vi "ElevatorManualControl.vi"(9 "Elevator State":string) -> (0 "Manual Contribution":dbl)   [LabVIEW 2018]
uses:
  Inputs_DriverStation.vi
  RobotStates.vi
panel:
  in  "Max Climb Down Power":dbl=0.2
  in  "Max Climb Up Power":dbl=0.6
  in  "Bump Up":dbl=1.0
  in  "Bump Down":dbl=1.0
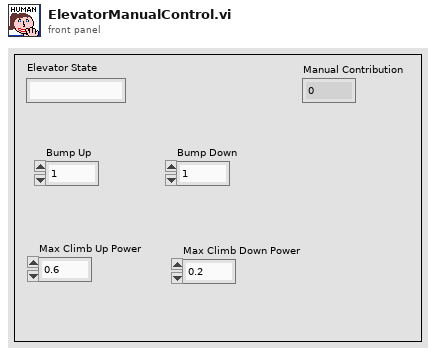
[diagram p1: front panel]
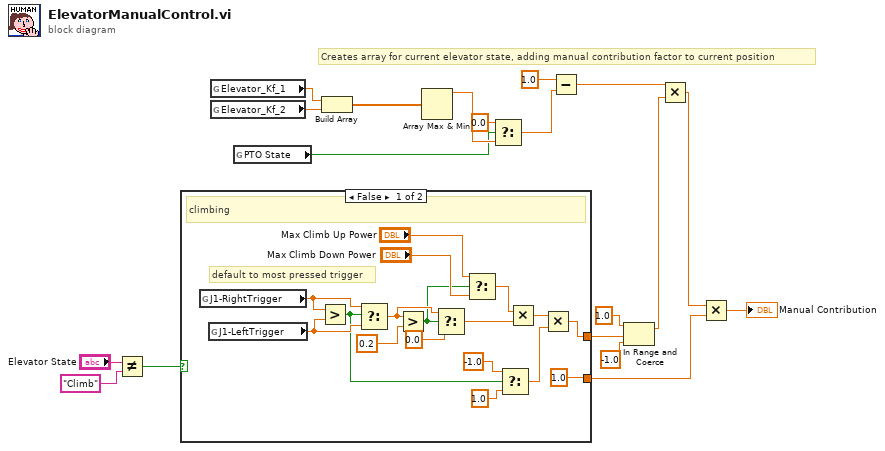
[diagram p0: block diagram]
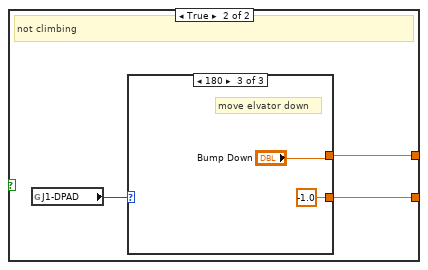
[diagram p2: hidden frame]
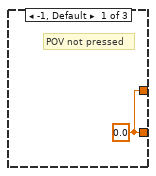
[diagram p3: hidden frame]
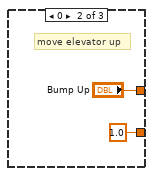
[diagram p4: hidden frame]
diagram:
  # "Creates array for current elevator state, adding manual contribution factor to current position"
  n1 = Not Equal?(x="Elevator State", y="Climb") -> (x != y?=w2:bool)
  n2 = case shown="False" w2 {
    tunnel: [1.0 w39] -> w19
    tunnel: [w23 w38] -> w12
    frame False {
      # "default to most pressed trigger"
      # "climbing"
      n3 = global read "Inputs_DriverStation.vi" "J1-RightTrigger"() -> (w36:dbl)
      n4 = global read "Inputs_DriverStation.vi" "J1-LeftTrigger"() -> (w35:dbl)
      n5 = Greater?(x=w36, y=w35) -> (0:w21:bool)
      n6 = Select(t=w36, s=w21, f=w35) -> (s? t:f=w33:dbl)
      n7 = Greater?(x=w33, y=0.2) -> (0:w27:bool)
      n8 = Select(t=w33, s=w27, f=0.0) -> (s? t:f=w30:dbl)
      n9 = Select(t="Max Climb Up Power", s=w27, f="Max Climb Down Power") -> (s? t:f=w31:dbl)
      n10 = Select(t=-1.0, s=w21, f=1.0) -> (s? t:f=w22:dbl)
      n11 = Multiply(x=w31, y=w30) -> (x*y=w24:dbl)
      n12 = Multiply(x=w24, y=w22) -> (x*y=w23:dbl)
    }
    frame True {
      # "not climbing"
      n13 = global read "Inputs_DriverStation.vi" "J1-DPAD"() -> (w37:i16)
      n14 = case shown="180" w37 {
        tunnel: [w40 1.0 -1.0] -> w39
        tunnel: [w40 "Bump Up" "Bump Down"] -> w38
        frame -1, Default {
          w40 = 0.0
          # "POV not pressed"
        }
        frame 0 {
          # "move elevator up"
        }
        frame 180 {
          # "move elvator down"
        }
      }
    }
  }
  n15 = global read "Inputs_DriverStation.vi" "Elevator_Kf_1"() -> (w11:dbl)
  n16 = global read "Inputs_DriverStation.vi" "Elevator_Kf_2"() -> (w10:dbl)
  n17 = global read "RobotStates.vi" "PTO State"() -> (w5:bool)
  n18 = Build Array(w11, w10) -> (w9:dbl[])
  n19 = Array Max & Min(array=w9) -> (max value=w8:dbl)  [unwired: 3 out]
  n20 = Select(t=0.0, s=w5, f=w8) -> (s? t:f=w7:dbl)
  n21 = Subtract(x=1.0, y=w7) -> (x-y=w17:dbl)
  n22 = In Range and Coerce(upper limit=1.0, x=w12, lower limit=-1.0) -> (coerced(x)=w13:dbl)  [unwired: 1 out]
  n23 = Multiply(x=w17, y=w13) -> (x*y=w16:dbl)
  n24 = Multiply(x=w16, y=w19) -> (x*y=→"Manual Contribution":dbl)
